vi "Flatten Header.vi"(11 "Header in":T1) -> (3 "Flattened Data out":u8[](array[numeric]) format="%.0x")   [LabVIEW 2021, in "ChannelCommon.lvlib"]
uses:
  ChannelCommon.lvlib
  <vilib>/CIF Foundation/CIF Utilities/DataTypes/DataTypes_CIF_U.lvlib
  typedef/FIFO Header.ctl
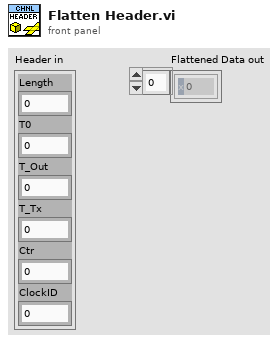
[diagram p1: front panel]
types:
  T1 = typedef "ChannelCommon.lvlib/FIFO Header.ctl" = cluster{"Length":u64, "T0":i64, "T_Out":i64, "T_Tx":i64, "Ctr":u64, "ClockID":u8}
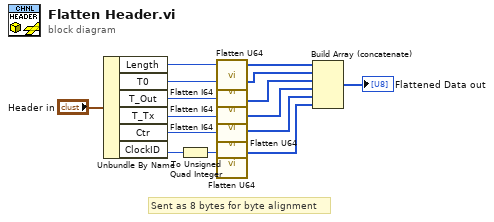
[diagram p0: block diagram]
diagram:
  # "Sent as 8 bytes for byte alignment"
  n1 = Unbundle By Name("Header in") -> ("Length"=w14:u64, "T0"=w13:i64, "T_Out"=w12:i64, "T_Tx"=w11:i64, "Ctr"=w10:u64, "ClockID"=w4:u8)
  n2 = To Unsigned Quad Integer(1:w4) -> (0:w3:u64)
  n3 = call <vilib>:"Flatten U64.vi"("U64"=w14) -> ("Flat Data"=w9:u8[])  [unwired: 4 in]
  n4 = call <vilib>:"Flatten I64.vi"("I64"=w13) -> ("Flat Data"=w8:u8[])  [unwired: 4 in]
  n5 = call <vilib>:"Flatten I64.vi"("I64"=w12) -> ("Flat Data"=w7:u8[])  [unwired: 4 in]
  n6 = call <vilib>:"Flatten I64.vi"("I64"=w11) -> ("Flat Data"=w6:u8[])  [unwired: 4 in]
  n7 = call <vilib>:"Flatten U64.vi"("U64"=w10) -> ("Flat Data"=w5:u8[])  [unwired: 4 in]
  n8 = call <vilib>:"Flatten U64.vi"("U64"=w3) -> ("Flat Data"=w2:u8[])  [unwired: 4 in]
  n9 = Build Array (concatenate)(w9, w8, w7, w6, w5, w2) -> (→"Flattened Data out":u8[])
